vi "Get Buffer Filling Mode.vi"(0 "VISA resource name":refnum<visa-resource-name>, 5 "Buffer Name (defbuffer1)":string, 11 "error in (no error)":errorcluster) -> (4 "VISA resource name out":refnum<visa-resource-name>, 8 "Fill Type":u16(ring) items=["Continuous", "Once"], 15 "error out":errorcluster)   [LabVIEW 2009, in "Keithley DMM7510.lvlib"]
doc: "This finds whether the reading buffer is filled continuously or is filled once and stops."
uses:
  Keithley DMM7510.lvlib
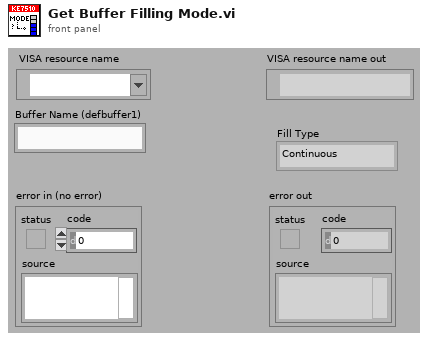
[diagram p1: front panel]
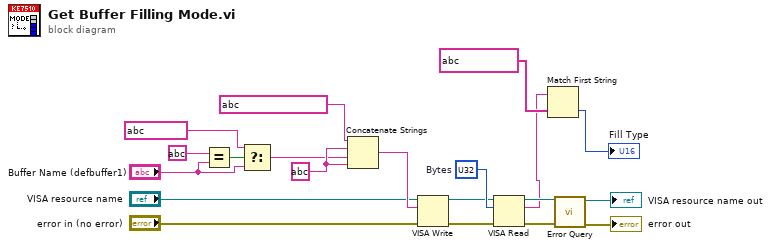
[diagram p0: block diagram]
diagram:
  w13 = string ?
  w17 = u32 ?  # Bytes
  n1 = Equal?(x=string ?, y="Buffer Name (defbuffer1)") -> (x = y?=w15:bool)
  n2 = Select(t=string ?, s=w15, f="Buffer Name (defbuffer1)") -> (s? t:f=w12:string)
  n3 = Concatenate Strings(string ? ("Fetch Measurement"), w13, w12, w13) -> (w18:string)
  n4 = VISA Write(VISA resource name="VISA resource name", write buffer=w18, error in (no error)="error in (no error)") -> (VISA resource name out=w8:refnum<visa-resource-name>, error out=w7:errorcluster)  [unwired: 1 out]
  n5 = VISA Read(VISA resource name=w8, byte count=w17, error in (no error)=w7) -> (VISA resource name out=w6:refnum<visa-resource-name>, read buffer=w1:string, error out=w5:errorcluster)  [unwired: 1 out]
  n6 = Match First String(2:string[] ?, 3:w1) -> (0:→"Fill Type":i32)  [unwired: 1 out]
  n7 = call "Error Query.vi"("error in (no error)"=w5, "VISA resource name"=w6) -> ("error out"=→"error out":errorcluster, "VISA resource name out"=→"VISA resource name out":refnum<visa-resource-name>)  [unwired: 8 out]
